vi "VL6180 GetDistance.vi"(6 "Speed Read":bool, 8 "error in (no error)":errorcluster, 9 "Attempts before Timeout":u16=10, 10 "VL6180 Resource in":T8 {"I2C Slave Address" format="%02x"}, 11 "LINX Resource":T2) -> (0 "error out":errorcluster, 1 "ToF Reading":T1, 2 "VL6180 Resource out":T8 {"I2C Slave Address" format="%02x"}, 3 "LINX Resource":T2, 4 "VL6180 Error":cluster{"Error Code":u8, "# attempts":i32})   [LabVIEW 2018]
uses:
  VL6180X DEFS.ctl
  VL6180 Resource.ctl
  <vilib>/MakerHub/LINX/Private/Type Defs/Platform.ctl
  <vilib>/MakerHub/LINX/Private/Type Defs/Interface.ctl
  <vilib>/MakerHub/LINX/Private/Device/Type Defs/TCP Config.ctl
  <vilib>/MakerHub/LINX/Private/Device/Type Defs/Channels.ctl
  <vilib>/MakerHub/LINX/Private/Device/Type Defs/LINX Device Config.ctl
  <vilib>/MakerHub/LINX/Private/Type Defs/LINX Ref.ctl
  Type Defs/tofReading.ctl
panel:
  # "0 = No error\n6 = early convergence estimate check failed\n7 = max convergence issue"
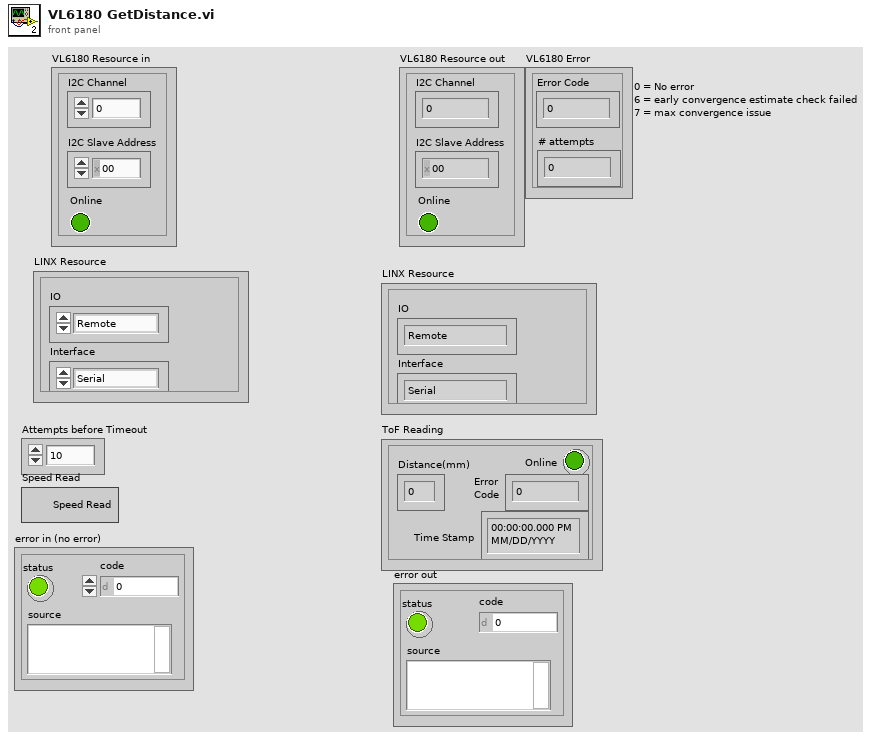
[diagram p1: front panel]
types:
  T1 = typedef "tofReading.ctl" = cluster{"Distance(mm)":u8, "Online":bool, "Error\nCode":u8, "Time Stamp":timestamp}
  T2 = typedef "LMH-LINX.lvlib/LINX Ref.ctl" = cluster{"IO":T3, "Interface":T4, "LINX Device Config":T5}
  T3 = typedef "LMH-LINX.lvlib/Platform.ctl" = enum16{"Remote", "Local"}
  T4 = typedef "LMH-LINX.lvlib/Interface.ctl" = enum16{"Serial", "TCP"}
  T5 = typedef "LMH-LINX.lvlib/Device.lvlib/LINX Device Config.ctl" = cluster{"Interface":T4, "COM Port":refnum<visa-resource-name>, "TCP Configuration":T6, "Device Family":u8, "Device ID":u8, "Device Name":string, "TCP Ref":refnum<k5>, "Channels":T7}
  T6 = typedef "LMH-LINX.lvlib/Device.lvlib/TCP Config.ctl" = cluster{"IP Address":string, "Port":u16}
  T7 = typedef "LMH-LINX.lvlib/Channels.ctl" = cluster{"DI":u8[], "DO":u8[], "AI":u8[], "AO":u8[], "PWM":u8[], "QE":u8[], "UART":u8[], "I2C 2":u8[], "SPI":u8[], "CAN":u8[], "Servo":u8[], "AI Ref (V)":dbl, "AI Resolution (Bits)":u8, "AO Ref (V)":dbl, "AO Resolution (Bits)":u8}
  T8 = typedef "VL6180 Resource.ctl" = cluster{"I2C Channel":u8, "I2C Slave Address":u8, "Online":bool}
  T9 = typedef "VL6180X DEFS.ctl" = u16
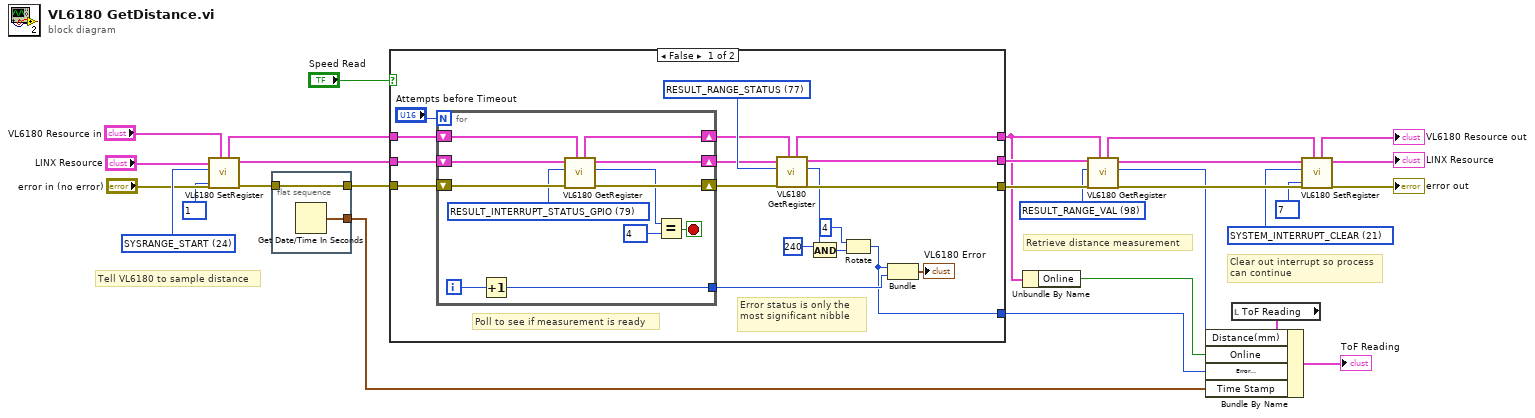
[diagram p0: block diagram]
diagram:
  w17 = T9 98 items=["IDENTIFICATION_MODEL_ID"=0, "IDENTIFICATION_MODEL_REV_MAJOR"=1, "IDENTIFICATION_MODEL_REV_MINOR"=2, "IDENTIFICATION_MODULE_REV_MAJOR"=3, "IDENTIFICATION_MODULE_REV_MINOR"=4, "IDENTIFICATION_DATE"=6, "IDENTIFICATION_TIME"=8, "SYSTEM_MODE_GPIO0"=16, "SYSTEM_MODE_GPIO1"=17, "SYSTEM_HISTORY_CTRL"=18, "SYSTEM_INTERRUPT_CONFIG_GPIO"=20, "SYSTEM_INTERRUPT_CLEAR"=21, "SYSTEM_FRESH_OUT_OF_RESET"=22, "SYSTEM_GROUPED_PARAMETER_HOLD"=23, "SYSRANGE_START"=24, "SYSRANGE_THRESH_HIGH"=25, "SYSRANGE_THRESH_LOW"=26, "SYSRANGE_INTERMEASUREMENT_PERIOD"=27, "SYSRANGE_MAX_CONVERGENCE_TIME"=28, "SYSRANGE_CROSSTALK_COMPENSATION_RATE"=30, "SYSRANGE_CROSSTALK_VALID_HEIGHT"=33, "SYSRANGE_EARLY_CONVERGENCE_ESTIMATE"=34, "SYSRANGE_PART_TO_PART_RANGE_OFFSET"=36, "SYSRANGE_RANGE_IGNORE_VALID_HEIGHT"=37, "SYSRANGE_RANGE_IGNORE_THRESHOLD"=38, "SYSRANGE_MAX_AMBIENT_LEVEL_MULT"=44, "SYSRANGE_RANGE_CHECK_ENABLES"=45, "SYSRANGE_VHV_RECALIBRATE"=46, "SYSRANGE_VHV_REPEAT_RATE"=49, "SYSALS_START"=56, "SYSALS_THRESH_HIGH"=58, "SYSALS_THRESH_LOW"=60, "SYSALS_INTERMEASUREMENT_PERIOD"=62, "SYSALS_ANALOGUE_GAIN"=63, "SYSALS_INTEGRATION_PERIOD"=64, "RESULT_RANGE_STATUS"=77, "RESULT_ALS_STATUS"=78, "RESULT_INTERRUPT_STATUS_GPIO"=79, "RESULT_ALS_VAL"=80, "RESULT_HISTORY_BUFFER"=82, "RESULT_RANGE_VAL"=98, "RESULT_RANGE_RAW"=100, "RESULT_RANGE_RETURN_RATE"=102, "RESULT_RANGE_REFERENCE_RATE"=104, "RESULT_RANGE_RETURN_SIGNAL_COUNT"=108, "RESULT_RANGE_REFERENCE_SIGNAL_COUNT"=112, "RESULT_RANGE_RETURN_AMB_COUNT"=116, "RESULT_RANGE_REFERENCE_AMB_COUNT"=120, "RESULT_RANGE_RETURN_CONV_TIME"=124, "RESULT_RANGE_REFERENCE_CONV_TIME"=128, "READOUT_AVERAGING_SAMPLE_PERIOD"=266, "FIRMWARE_BOOTUP"=281, "FIRMWARE_RESULT_SCALER"=288, "I2C_SLAVE_DEVICE_ADDRESS"=530, "INTERLEAVED_MODE_ENABLE"=675] ("Address")
  w21 = T9 21 items=["IDENTIFICATION_MODEL_ID"=0, "IDENTIFICATION_MODEL_REV_MAJOR"=1, "IDENTIFICATION_MODEL_REV_MINOR"=2, "IDENTIFICATION_MODULE_REV_MAJOR"=3, "IDENTIFICATION_MODULE_REV_MINOR"=4, "IDENTIFICATION_DATE"=6, "IDENTIFICATION_TIME"=8, "SYSTEM_MODE_GPIO0"=16, "SYSTEM_MODE_GPIO1"=17, "SYSTEM_HISTORY_CTRL"=18, "SYSTEM_INTERRUPT_CONFIG_GPIO"=20, "SYSTEM_INTERRUPT_CLEAR"=21, "SYSTEM_FRESH_OUT_OF_RESET"=22, "SYSTEM_GROUPED_PARAMETER_HOLD"=23, "SYSRANGE_START"=24, "SYSRANGE_THRESH_HIGH"=25, "SYSRANGE_THRESH_LOW"=26, "SYSRANGE_INTERMEASUREMENT_PERIOD"=27, "SYSRANGE_MAX_CONVERGENCE_TIME"=28, "SYSRANGE_CROSSTALK_COMPENSATION_RATE"=30, "SYSRANGE_CROSSTALK_VALID_HEIGHT"=33, "SYSRANGE_EARLY_CONVERGENCE_ESTIMATE"=34, "SYSRANGE_PART_TO_PART_RANGE_OFFSET"=36, "SYSRANGE_RANGE_IGNORE_VALID_HEIGHT"=37, "SYSRANGE_RANGE_IGNORE_THRESHOLD"=38, "SYSRANGE_MAX_AMBIENT_LEVEL_MULT"=44, "SYSRANGE_RANGE_CHECK_ENABLES"=45, "SYSRANGE_VHV_RECALIBRATE"=46, "SYSRANGE_VHV_REPEAT_RATE"=49, "SYSALS_START"=56, "SYSALS_THRESH_HIGH"=58, "SYSALS_THRESH_LOW"=60, "SYSALS_INTERMEASUREMENT_PERIOD"=62, "SYSALS_ANALOGUE_GAIN"=63, "SYSALS_INTEGRATION_PERIOD"=64, "RESULT_RANGE_STATUS"=77, "RESULT_ALS_STATUS"=78, "RESULT_INTERRUPT_STATUS_GPIO"=79, "RESULT_ALS_VAL"=80, "RESULT_HISTORY_BUFFER"=82, "RESULT_RANGE_VAL"=98, "RESULT_RANGE_RAW"=100, "RESULT_RANGE_RETURN_RATE"=102, "RESULT_RANGE_REFERENCE_RATE"=104, "RESULT_RANGE_RETURN_SIGNAL_COUNT"=108, "RESULT_RANGE_REFERENCE_SIGNAL_COUNT"=112, "RESULT_RANGE_RETURN_AMB_COUNT"=116, "RESULT_RANGE_REFERENCE_AMB_COUNT"=120, "RESULT_RANGE_RETURN_CONV_TIME"=124, "RESULT_RANGE_REFERENCE_CONV_TIME"=128, "READOUT_AVERAGING_SAMPLE_PERIOD"=266, "FIRMWARE_BOOTUP"=281, "FIRMWARE_RESULT_SCALER"=288, "I2C_SLAVE_DEVICE_ADDRESS"=530, "INTERLEAVED_MODE_ENABLE"=675] ("Address")
  w26 = T9 24 items=["IDENTIFICATION_MODEL_ID"=0, "IDENTIFICATION_MODEL_REV_MAJOR"=1, "IDENTIFICATION_MODEL_REV_MINOR"=2, "IDENTIFICATION_MODULE_REV_MAJOR"=3, "IDENTIFICATION_MODULE_REV_MINOR"=4, "IDENTIFICATION_DATE"=6, "IDENTIFICATION_TIME"=8, "SYSTEM_MODE_GPIO0"=16, "SYSTEM_MODE_GPIO1"=17, "SYSTEM_HISTORY_CTRL"=18, "SYSTEM_INTERRUPT_CONFIG_GPIO"=20, "SYSTEM_INTERRUPT_CLEAR"=21, "SYSTEM_FRESH_OUT_OF_RESET"=22, "SYSTEM_GROUPED_PARAMETER_HOLD"=23, "SYSRANGE_START"=24, "SYSRANGE_THRESH_HIGH"=25, "SYSRANGE_THRESH_LOW"=26, "SYSRANGE_INTERMEASUREMENT_PERIOD"=27, "SYSRANGE_MAX_CONVERGENCE_TIME"=28, "SYSRANGE_CROSSTALK_COMPENSATION_RATE"=30, "SYSRANGE_CROSSTALK_VALID_HEIGHT"=33, "SYSRANGE_EARLY_CONVERGENCE_ESTIMATE"=34, "SYSRANGE_PART_TO_PART_RANGE_OFFSET"=36, "SYSRANGE_RANGE_IGNORE_VALID_HEIGHT"=37, "SYSRANGE_RANGE_IGNORE_THRESHOLD"=38, "SYSRANGE_MAX_AMBIENT_LEVEL_MULT"=44, "SYSRANGE_RANGE_CHECK_ENABLES"=45, "SYSRANGE_VHV_RECALIBRATE"=46, "SYSRANGE_VHV_REPEAT_RATE"=49, "SYSALS_START"=56, "SYSALS_THRESH_HIGH"=58, "SYSALS_THRESH_LOW"=60, "SYSALS_INTERMEASUREMENT_PERIOD"=62, "SYSALS_ANALOGUE_GAIN"=63, "SYSALS_INTEGRATION_PERIOD"=64, "RESULT_RANGE_STATUS"=77, "RESULT_ALS_STATUS"=78, "RESULT_INTERRUPT_STATUS_GPIO"=79, "RESULT_ALS_VAL"=80, "RESULT_HISTORY_BUFFER"=82, "RESULT_RANGE_VAL"=98, "RESULT_RANGE_RAW"=100, "RESULT_RANGE_RETURN_RATE"=102, "RESULT_RANGE_REFERENCE_RATE"=104, "RESULT_RANGE_RETURN_SIGNAL_COUNT"=108, "RESULT_RANGE_REFERENCE_SIGNAL_COUNT"=112, "RESULT_RANGE_RETURN_AMB_COUNT"=116, "RESULT_RANGE_REFERENCE_AMB_COUNT"=120, "RESULT_RANGE_RETURN_CONV_TIME"=124, "RESULT_RANGE_REFERENCE_CONV_TIME"=128, "READOUT_AVERAGING_SAMPLE_PERIOD"=266, "FIRMWARE_BOOTUP"=281, "FIRMWARE_RESULT_SCALER"=288, "I2C_SLAVE_DEVICE_ADDRESS"=530, "INTERLEAVED_MODE_ENABLE"=675] ("Address")
  # "Retrieve distance measurement"
  # "Tell VL6180 to sample distance"
  # "Clear out interrupt so process can continue"
  n1 = call "VL6180 SetRegister.vi"("VL6180 Resource"="VL6180 Resource in", "error in (no error)"="error in (no error)", "Data in"=u8 1, "Address"=w26, "LINX Resource"="LINX Resource") -> ("error out"=w8:errorcluster, "LINX Resource"=w25:T2, "VL6180 Resource"=w11:T8)  [unwired: 4 in]
  n2 = flat-sequence {
    tunnel: w8 -> [w30]
    tunnel: [w30] -> w7
    tunnel: [w29] -> w1
    frame #0 {
      n3 = Get Date/Time In Seconds() -> (seconds since 1Jan1904=w29:timestamp)
    }
  }
  n4 = case shown="False" "Speed Read" {
    tunnel: [w48 w61] -> w28
    tunnel: [w47 w62] -> w27
    tunnel: w7 -> [w46 w61]
    tunnel: w25 -> [w45 w62]
    tunnel: [w44 w63] -> w3
    tunnel: w11 -> [w43 w63]
    tunnel: [w31 _] -> w5
    frame False {
      w38 = T9 77 items=["IDENTIFICATION_MODEL_ID"=0, "IDENTIFICATION_MODEL_REV_MAJOR"=1, "IDENTIFICATION_MODEL_REV_MINOR"=2, "IDENTIFICATION_MODULE_REV_MAJOR"=3, "IDENTIFICATION_MODULE_REV_MINOR"=4, "IDENTIFICATION_DATE"=6, "IDENTIFICATION_TIME"=8, "SYSTEM_MODE_GPIO0"=16, "SYSTEM_MODE_GPIO1"=17, "SYSTEM_HISTORY_CTRL"=18, "SYSTEM_INTERRUPT_CONFIG_GPIO"=20, "SYSTEM_INTERRUPT_CLEAR"=21, "SYSTEM_FRESH_OUT_OF_RESET"=22, "SYSTEM_GROUPED_PARAMETER_HOLD"=23, "SYSRANGE_START"=24, "SYSRANGE_THRESH_HIGH"=25, "SYSRANGE_THRESH_LOW"=26, "SYSRANGE_INTERMEASUREMENT_PERIOD"=27, "SYSRANGE_MAX_CONVERGENCE_TIME"=28, "SYSRANGE_CROSSTALK_COMPENSATION_RATE"=30, "SYSRANGE_CROSSTALK_VALID_HEIGHT"=33, "SYSRANGE_EARLY_CONVERGENCE_ESTIMATE"=34, "SYSRANGE_PART_TO_PART_RANGE_OFFSET"=36, "SYSRANGE_RANGE_IGNORE_VALID_HEIGHT"=37, "SYSRANGE_RANGE_IGNORE_THRESHOLD"=38, "SYSRANGE_MAX_AMBIENT_LEVEL_MULT"=44, "SYSRANGE_RANGE_CHECK_ENABLES"=45, "SYSRANGE_VHV_RECALIBRATE"=46, "SYSRANGE_VHV_REPEAT_RATE"=49, "SYSALS_START"=56, "SYSALS_THRESH_HIGH"=58, "SYSALS_THRESH_LOW"=60, "SYSALS_INTERMEASUREMENT_PERIOD"=62, "SYSALS_ANALOGUE_GAIN"=63, "SYSALS_INTEGRATION_PERIOD"=64, "RESULT_RANGE_STATUS"=77, "RESULT_ALS_STATUS"=78, "RESULT_INTERRUPT_STATUS_GPIO"=79, "RESULT_ALS_VAL"=80, "RESULT_HISTORY_BUFFER"=82, "RESULT_RANGE_VAL"=98, "RESULT_RANGE_RAW"=100, "RESULT_RANGE_RETURN_RATE"=102, "RESULT_RANGE_REFERENCE_RATE"=104, "RESULT_RANGE_RETURN_SIGNAL_COUNT"=108, "RESULT_RANGE_REFERENCE_SIGNAL_COUNT"=112, "RESULT_RANGE_RETURN_AMB_COUNT"=116, "RESULT_RANGE_REFERENCE_AMB_COUNT"=120, "RESULT_RANGE_RETURN_CONV_TIME"=124, "RESULT_RANGE_REFERENCE_CONV_TIME"=128, "READOUT_AVERAGING_SAMPLE_PERIOD"=266, "FIRMWARE_BOOTUP"=281, "FIRMWARE_RESULT_SCALER"=288, "I2C_SLAVE_DEVICE_ADDRESS"=530, "INTERLEAVED_MODE_ENABLE"=675] ("Address")
      # "Poll to see if measurement is ready"
      # "Error status is only the most significant nibble"
      n5 = for {
        N: "Attempts before Timeout" -> [_]
        shift-right: [w58] -> w36
        shift-left: w45 -> [w60]
        shift-right: [w57] -> w37
        shift-left: w46 -> [w59]
        shift-right: [w51] -> w35
        shift-left: w43 -> [w52]
        tunnel: [w49] -> w33
        i -> [w50]
        stop <- w53 stop-if-true
        w54 = T9 79 items=["IDENTIFICATION_MODEL_ID"=0, "IDENTIFICATION_MODEL_REV_MAJOR"=1, "IDENTIFICATION_MODEL_REV_MINOR"=2, "IDENTIFICATION_MODULE_REV_MAJOR"=3, "IDENTIFICATION_MODULE_REV_MINOR"=4, "IDENTIFICATION_DATE"=6, "IDENTIFICATION_TIME"=8, "SYSTEM_MODE_GPIO0"=16, "SYSTEM_MODE_GPIO1"=17, "SYSTEM_HISTORY_CTRL"=18, "SYSTEM_INTERRUPT_CONFIG_GPIO"=20, "SYSTEM_INTERRUPT_CLEAR"=21, "SYSTEM_FRESH_OUT_OF_RESET"=22, "SYSTEM_GROUPED_PARAMETER_HOLD"=23, "SYSRANGE_START"=24, "SYSRANGE_THRESH_HIGH"=25, "SYSRANGE_THRESH_LOW"=26, "SYSRANGE_INTERMEASUREMENT_PERIOD"=27, "SYSRANGE_MAX_CONVERGENCE_TIME"=28, "SYSRANGE_CROSSTALK_COMPENSATION_RATE"=30, "SYSRANGE_CROSSTALK_VALID_HEIGHT"=33, "SYSRANGE_EARLY_CONVERGENCE_ESTIMATE"=34, "SYSRANGE_PART_TO_PART_RANGE_OFFSET"=36, "SYSRANGE_RANGE_IGNORE_VALID_HEIGHT"=37, "SYSRANGE_RANGE_IGNORE_THRESHOLD"=38, "SYSRANGE_MAX_AMBIENT_LEVEL_MULT"=44, "SYSRANGE_RANGE_CHECK_ENABLES"=45, "SYSRANGE_VHV_RECALIBRATE"=46, "SYSRANGE_VHV_REPEAT_RATE"=49, "SYSALS_START"=56, "SYSALS_THRESH_HIGH"=58, "SYSALS_THRESH_LOW"=60, "SYSALS_INTERMEASUREMENT_PERIOD"=62, "SYSALS_ANALOGUE_GAIN"=63, "SYSALS_INTEGRATION_PERIOD"=64, "RESULT_RANGE_STATUS"=77, "RESULT_ALS_STATUS"=78, "RESULT_INTERRUPT_STATUS_GPIO"=79, "RESULT_ALS_VAL"=80, "RESULT_HISTORY_BUFFER"=82, "RESULT_RANGE_VAL"=98, "RESULT_RANGE_RAW"=100, "RESULT_RANGE_RETURN_RATE"=102, "RESULT_RANGE_REFERENCE_RATE"=104, "RESULT_RANGE_RETURN_SIGNAL_COUNT"=108, "RESULT_RANGE_REFERENCE_SIGNAL_COUNT"=112, "RESULT_RANGE_RETURN_AMB_COUNT"=116, "RESULT_RANGE_REFERENCE_AMB_COUNT"=120, "RESULT_RANGE_RETURN_CONV_TIME"=124, "RESULT_RANGE_REFERENCE_CONV_TIME"=128, "READOUT_AVERAGING_SAMPLE_PERIOD"=266, "FIRMWARE_BOOTUP"=281, "FIRMWARE_RESULT_SCALER"=288, "I2C_SLAVE_DEVICE_ADDRESS"=530, "INTERLEAVED_MODE_ENABLE"=675] ("Address")
        n6 = Increment(x=w50) -> (x+1=w49:i32)
        n7 = call "VL6180 GetRegister.vi"("VL6180 Resource"=w52, "error in"=w59, "VL6180X Constants"=w54, "LINX Resource"=w60) -> ("error out"=w57:errorcluster, "Data out"=w55:u8, "LINX Resource"=w58:T2, "VL6180 Resource"=w51:T8)  [unwired: 4 in]
        n8 = Equal?(x=w55, y=u8 4 ("Data in")) -> (x = y?=w53:bool)
      }
      n9 = call "VL6180 GetRegister.vi"("VL6180 Resource"=w35, "error in"=w37, "VL6180X Constants"=w38, "LINX Resource"=w36) -> ("error out"=w48:errorcluster, "Data out"=w39:u8, "LINX Resource"=w47:T2, "VL6180 Resource"=w44:T8)  [unwired: 4 in]
      n10 = And(x=u8 240, y=w39) -> (x .and. y?=w41:u8)
      n11 = Rotate(1:w41, 2:i16 4 ("y")) -> (0:w31:u8)
      n12 = Bundle(w31, w33) -> (→"VL6180 Error":cluster{u8, i32})  [unwired: 1 in]
    }
    frame True {
    }
  }
  n13 = Unbundle By Name(w3) -> ("Online"=w2:bool)
  n14 = call "VL6180 GetRegister.vi"("VL6180 Resource"=w3, "error in"=w28, "VL6180X Constants"=w17, "LINX Resource"=w27) -> ("error out"=w24:errorcluster, "Data out"=w4:u8, "LINX Resource"=w22:T2, "VL6180 Resource"=w12:T8)  [unwired: 4 in]
  n15 = local read "ToF Reading"() -> (w9:T1)
  n16 = Bundle By Name(cluster=w9, "Distance(mm)"=w4, "Online"=w2, "Error\nCode"=w5, "Time Stamp"=w1) -> (→"ToF Reading":T1)
  n17 = call "VL6180 SetRegister.vi"("VL6180 Resource"=w12, "error in (no error)"=w24, "Data in"=u8 7, "Address"=w21, "LINX Resource"=w22) -> ("error out"=→"error out":errorcluster, "LINX Resource"=→"LINX Resource":T2, "VL6180 Resource"=→"VL6180 Resource out":T8)  [unwired: 4 in]
